vi "OPC UA Read.vi"() -> ()   [LabVIEW 2019]
uses:
  <vilib>/OPCUA/client/Multiple Read Double.vi
  <vilib>/OPCUA/NI OPC UA Client.lvlib
panel:
  out "resulting string":string
  out "Temperature":dbl
  in  "Node ID":string="ns=2;s=Temperature"
  in  "stop":bool
  in  "Server Endpoint URL":string="opc.tcp://LAPTOP-UEHKTQQC:49580"
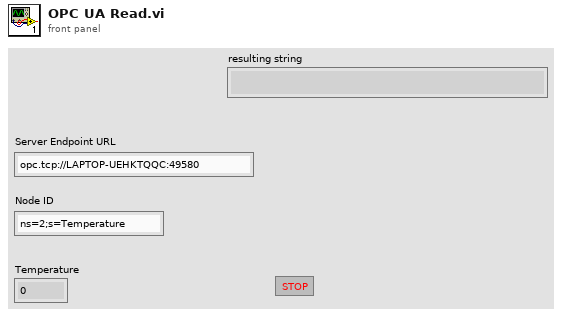
[diagram p1: front panel]
types:
  T1 = cluster{"message mode":enum16{"None", "Sign", "Sign and Encrypt"}, "security":enum16{"Basic256", "Basic128Rsa15"}}
  T2 = typedef "OPC UA Client Refnum.ctl" = refnum<k21>
  T3 = typedef "NodeId.ctl" = string
  T4 = typedef "OPC UA StatusCode.ctl" = u32
  T5 = cluster{"node ID":T3, "value ":dbl, "timestamp":timestamp, "status":T4}[]
  T6 = cluster{"node ID":T3, "value ":dbl, "timestamp":timestamp, "status":T4}
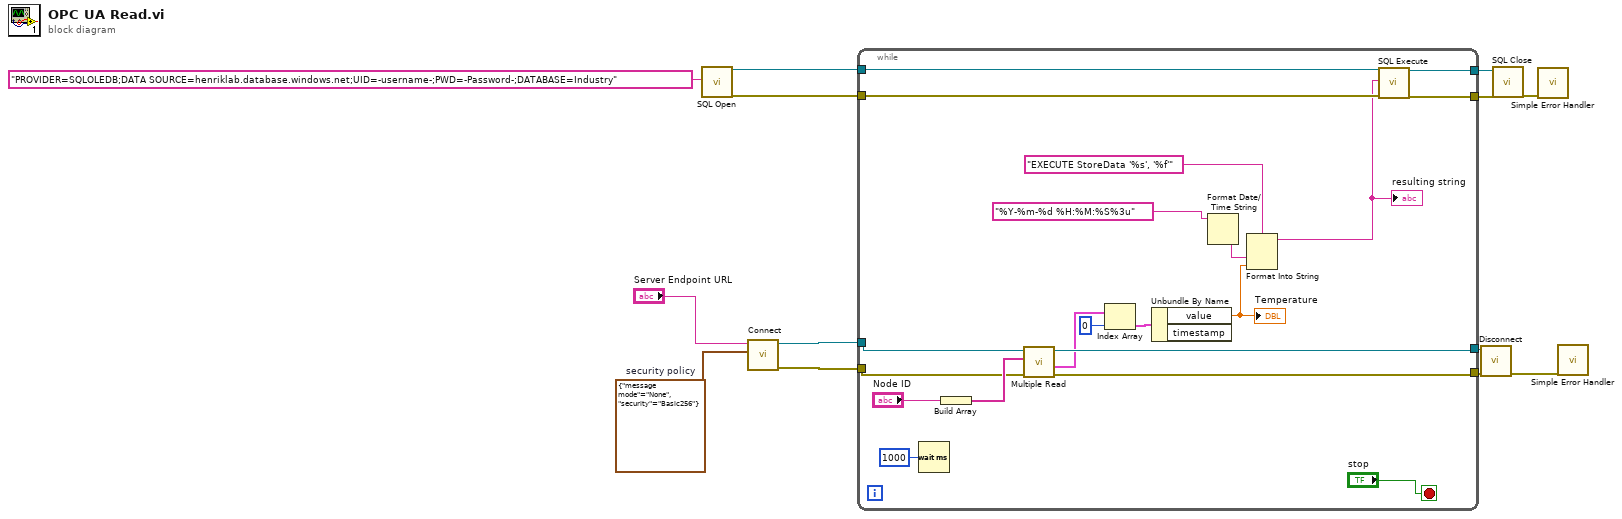
[diagram p0: block diagram]
diagram:
  w12 = T1 {"message mode"=enum."None", "security"=enum."Basic256"}  # security policy
  n1 = call <vilib>:"SQL Open.vi"("ConnectionString In"="PROVIDER=SQLOLEDB;DATA SOURCE=henriklab.database.windows.net;UID=-username-;PWD=-Password-;DATABASE=Industry") -> ("Connection Out"=w6:refnum<k7>, "Error out"=w4:errorcluster)  [unwired: 17 in]
  n2 = call <vilib>:"Connect.vi"("security policy"=w12, "server endpoint URL"="Server Endpoint URL") -> ("error out"=w10:errorcluster, "OPC UA client refnum out"=w11:T2)  [unwired: 7 in, 1 out]
  n3 = while {
    tunnel: w11 -> [w31]
    tunnel: w10 -> [w28]
    tunnel: [w27] -> w9
    tunnel: [w26] -> w8
    tunnel: w6 -> [w22]
    tunnel: [w21] -> w5
    tunnel: w4 -> [w20]
    tunnel: [w19] -> w3
    stop <- "stop" stop-if-true
    n4 = Wait (ms)(milliseconds to wait=u32 1000) -> ()  [unwired: 1 out]
    n5 = Build Array("Node ID") -> (w29:string[])
    n6 = call-poly <vilib>:"Multiple Read.vi"("error in (no error)"=w28, "node IDs"=w29, "OPC UA client refnum in"=w31) -> ("error out"=w26:errorcluster, "results"=w25:T5, "OPC UA client refnum out"=w27:T2)  [unwired: 5 in, 1 out]
    n7 = Index Array(array=w25, index=0) -> (element=w23:T6)
    n8 = Unbundle By Name(w23) -> ("value"=w17:dbl)  [unwired: 1 out]
    "Temperature" <- w17
    n9 = Format Date/Time String(time format string (%c)="%Y-%m-%d %H:%M:%S%3u") -> (date/time string=w18:string)  [unwired: 2 in]
    n10 = Format Into String "Format Into String"(format string="EXECUTE StoreData '%s', '%f'", w18, w17) -> (resulting string=w14:string)  [unwired: 2 in, 1 out]
    "resulting string" <- w14
    n11 = call <vilib>:"SQL Execute.vi"("Connection In"=w22, "SQL Query"=w14, "Error in (no error)"=w20) -> ("Connection Out"=w21:refnum<k7>, "Error out"=w19:errorcluster)  [unwired: 15 in]
  }
  n12 = call <vilib>:"Disconnect.vi"("error in (no error)"=w8, "OPC UA client refnum in"=w9) -> ("error out"=w7:errorcluster)  [unwired: 9 in]
  n13 = call <vilib>:"SQL Close.vi"("Connection In"=w5, "Error in (no error)"=w3) -> ("Error out"=w1:errorcluster)  [unwired: 17 in]
  n14 = call <vilib>:"Simple Error Handler.vi"("error in (no error)"=w1) -> ()  [unwired: 4 in, 5 out]
  n15 = call <vilib>:"Simple Error Handler.vi"("error in (no error)"=w7) -> ()  [unwired: 4 in, 5 out]
